vi "ex9.vi"() -> ()   [LabVIEW 2022 SP3]
panel:
  in  "Lower limit":dbl(knob) scale=0.0..1000.0
  in  "Upper limit":dbl(knob) scale=0.0..1000.0
  out "Number in range?":bool
  in  "Temp":dbl(slide) scale=0.0..1000.0
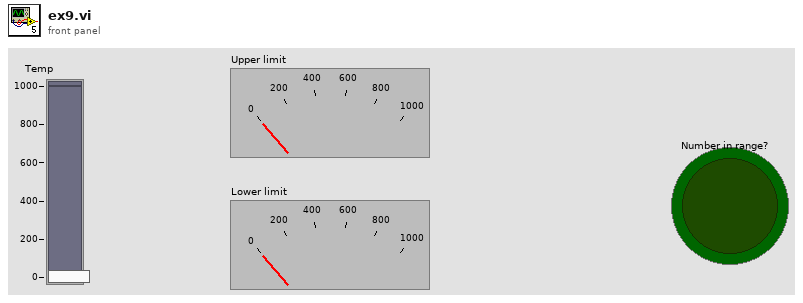
[diagram p1: front panel]
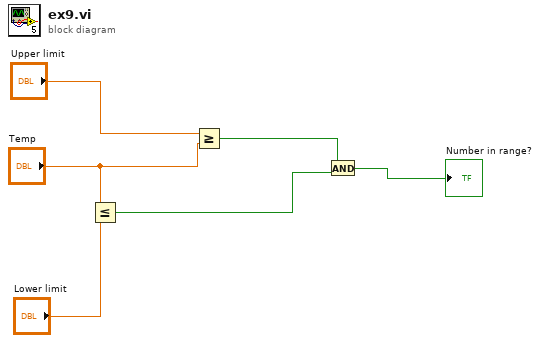
[diagram p0: block diagram]
diagram:
  n1 = Less Or Equal?(x="Lower limit", y="Temp") -> (x <= y?=w3:bool)
  n2 = Greater Or Equal?(x="Upper limit", y="Temp") -> (x >= y?=w4:bool)
  n3 = And(x=w4, y=w3) -> (x .and. y?=→"Number in range?":bool)
